vi "Barcode Scanner for ISN.vi"(9 "Please Scan ISN":string) -> (0 "Scan ok?":bool, 3 "String Indicator":string)   [LabVIEW 2017]
panel:
  out "当前长度":i32
  in  "stop":bool
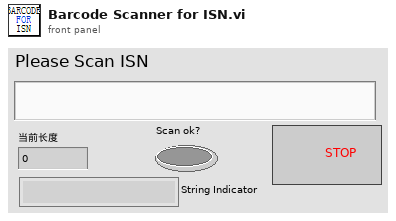
[diagram p1: front panel]
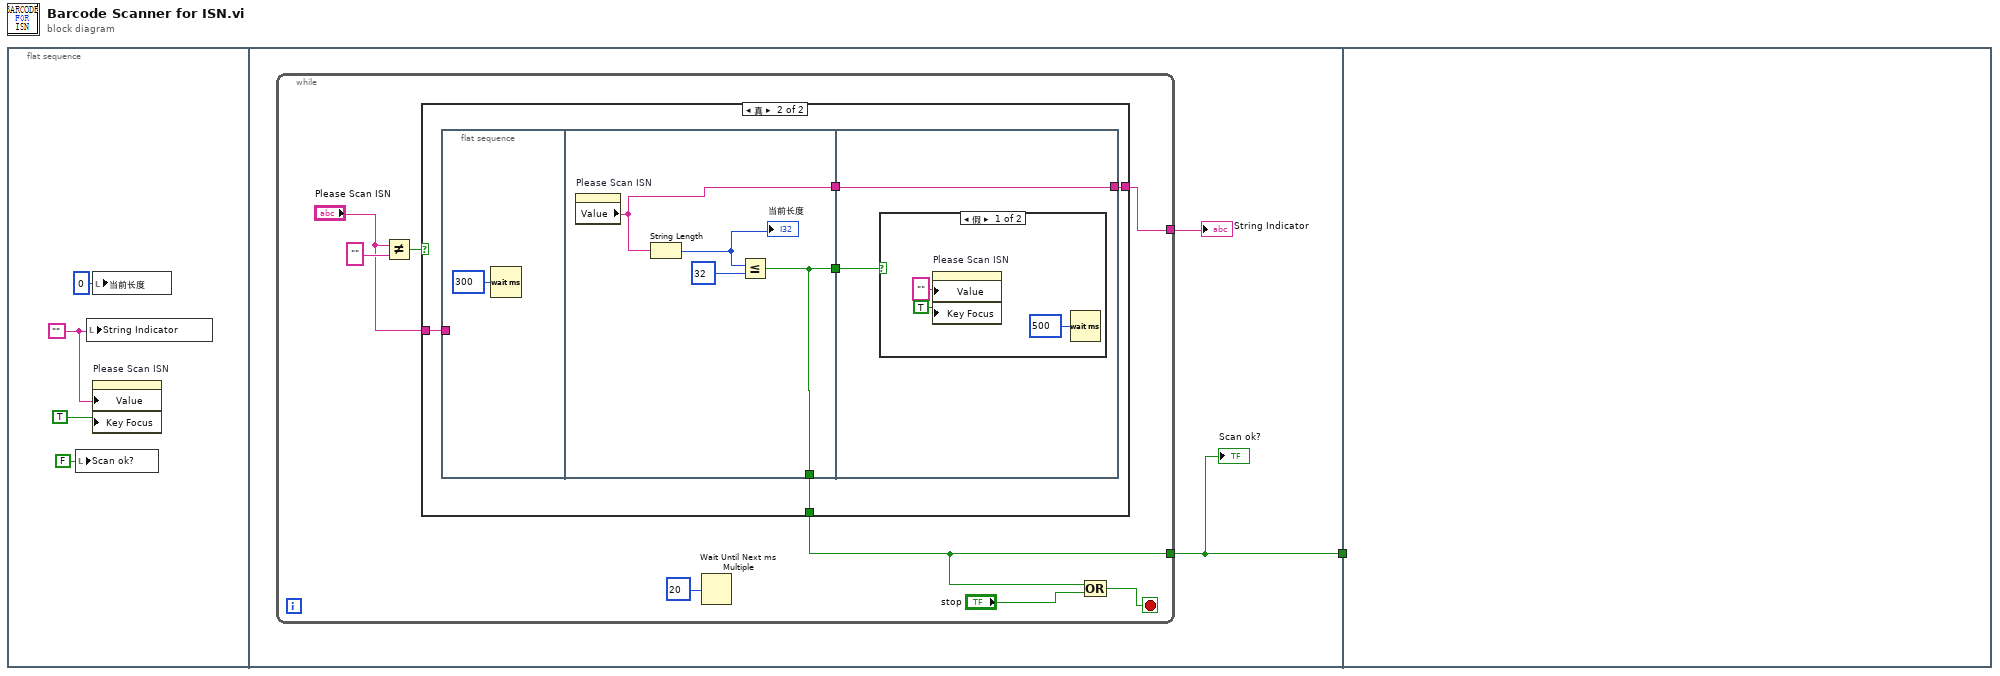
[diagram p0: block diagram]
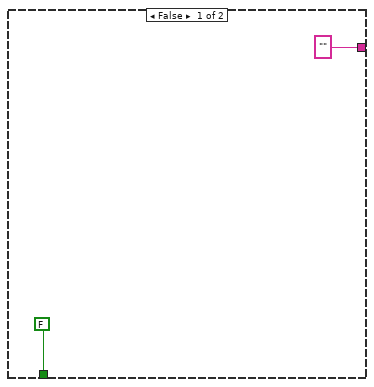
[diagram p2: hidden frame]
diagram:
  n1 = flat-sequence {
    tunnel: [w6] -> w1
    tunnel: w1 -> [_]
    frame #0 {
      w2 = ""
      n2 = local write "Scan ok?"(FALSE ("Scan ok?")) -> ()
      n3 = local write "String Indicator"(w2) -> ()
      n4 = local write "当前长度"(0 ("当前长度")) -> ()
      n5 = property on="Please Scan ISN" class="Str"("Value"=w2, "Key Focus"=TRUE ("键选中")) -> ()  [unwired: 2 in, 2 out]
    }
    frame #1 {
      n6 = while {
        tunnel: [w10] -> w7
        tunnel: [w9] -> w6
        stop <- w15 stop-if-true
        n7 = Not Equal?(x="Please Scan ISN", y="" ("Scan User ID")) -> (x != y?=w11:bool)
        n8 = case shown="真" w11 {
          tunnel: ["" ("Scan User ID") w20] -> w10
          tunnel: [FALSE w19] -> w9
          tunnel: "Please Scan ISN" -> [_ w18]
          frame False {
          }
          frame True {
            n9 = flat-sequence {
              tunnel: w18 -> [_]
              tunnel: [w25] -> w22
              tunnel: [w24] -> w21
              tunnel: [w25] -> w19
              tunnel: w22 -> [w29]
              tunnel: w21 -> [w28]
              tunnel: [w28] -> w20
              frame #0 {
                n10 = Wait (ms)(milliseconds to wait=u32 300 ("等待时间（毫秒）")) -> ()  [unwired: 1 out]
              }
              frame #1 {
                n11 = property on="Please Scan ISN" class="Str"() -> ("Value"=w24:string)  [unwired: 2 in, 2 out]
                n12 = String Length(string=w24) -> (length=w26:i32)
                "当前长度" <- w26
                n13 = Less Or Equal?(x=w26, y=32 ("长度")) -> (x <= y?=w25:bool)
              }
              frame #2 {
                n14 = case shown="假" w29 {
                  frame False {
                    n15 = property on="Please Scan ISN" class="Str"("Value"="" ("Scan User ID"), "Key Focus"=TRUE) -> ()  [unwired: 2 in, 2 out]
                    n16 = Wait (ms)(milliseconds to wait=u32 500 ("millisecond multiple")) -> ()  [unwired: 1 out]
                  }
                  frame True {
                  }
                }
              }
            }
          }
        }
        n17 = Wait Until Next ms Multiple(millisecond multiple=u32 20) -> ()  [unwired: 1 out]
        n18 = Compound Arithmetic op=OR(w9, "stop") -> (w15:bool)
      }
      "String Indicator" <- w7
      "Scan ok?" <- w6
    }
    frame #2 {
    }
  }
